vi "Preset Distance Vison Shots.vi"(10 "Distance":dbl) -> (2 "Hood Down?":bool, 3 "Shooter RPM":dbl)   [LabVIEW 2016]
uses:
  Robot Global Data.vi
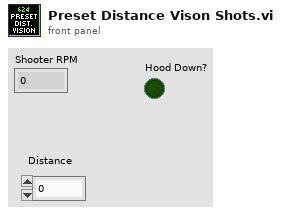
[diagram p1: front panel]
types:
  T1 = typedef "NI_Matrix.lvlib/RealMatrix.ctl" = dbl[][]
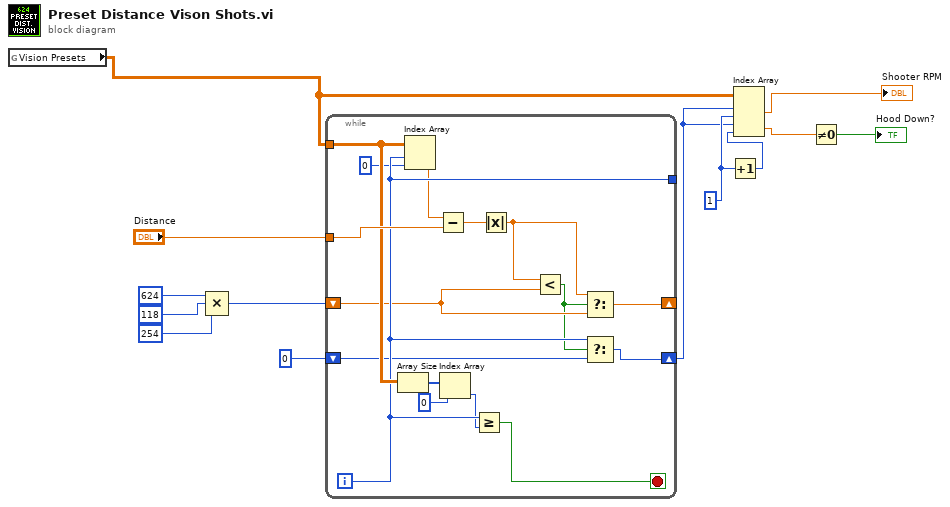
[diagram p0: block diagram]
diagram:
  w6 = 1 ("disabled index (col)")
  n1 = global read "Robot Global Data.vi" "Vision Presets"() -> (w4:T1)
  n2 = Compound Arithmetic op=MULTIPLY(624, 118 ("value"), 254 ("value")) -> (w8:i32)
  n3 = while {
    tunnel: "Distance" -> [w29]
    tunnel: w4 -> [w28]
    tunnel: [w26] -> _
    shift-right: [w24] -> _
    shift-left: w8 -> [w25]
    shift-right: [w22] -> w5
    shift-left: 0 -> [w23]
    i -> [w26]
    stop <- w27 stop-if-true
    n4 = Array Size(array=w28) -> (size(s)=w16:i32[])
    n5 = Index Array(array=w28, index (row)=w26, index (col)=0 ("disabled index (col)")) -> (element=w18:dbl)
    n6 = Subtract(x=w18, y=w29) -> (x-y=w21:dbl)
    n7 = Index Array(array=w16, index=0) -> (element=w14:i32)
    n8 = Greater Or Equal?(x=w26, y=w14) -> (x >= y?=w27:bool)
    n9 = Absolute Value(x=w21) -> (abs(x)=w20:dbl)
    n10 = Less?(x=w20, y=w25) -> (x < y?=w17:bool)
    n11 = Select(t=w20, s=w17, f=w25) -> (s? t:f=w24:dbl)
    n12 = Select(t=w26, s=w17, f=w23) -> (s? t:f=w22:i32)
  }
  n13 = Increment(x=w6) -> (x+1=w12:i32)
  n14 = Index Array(array=w4, index (row) #1=w5, index (col) #1=w6, index (row) #2=w5, index (col) #2=w12) -> (element #1=→"Shooter RPM":dbl, element #2=w3:dbl)
  n15 = Not Equal To 0?(x=w3) -> (x != 0?=→"Hood Down?":bool)
